vi "Configure Output.vi"(7 "Source Condition (2: Normal)":i32(ring)=2 items=["Zero", "HIZ", "Normal"], 8 "error in (no error)":errorcluster, 9 "Low Terminal State (1: Float)":i32(ring)=1 items=["Common", "Float"], 10 "Channel (1: Channel 1)":i32(ring)=1 items=["Channel 1"=1, "Channel 2"=2], 11 "VISA resource name":refnum<visa-resource-name>) -> (0 "error out":errorcluster, 3 "VISA resource name out":refnum<visa-resource-name>)   [LabVIEW 2017, in "Keysight B2980 Series.lvlib"]
doc: "Configures the low terminal and source condition for output.\n\n<b>Note(s):</b>\nThis VI is only applicable for model B2985A and B2987A."
uses:
  Keysight B2980 Series.lvlib
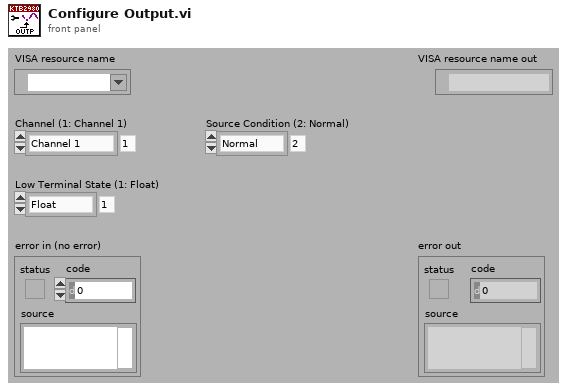
[diagram p1: front panel]
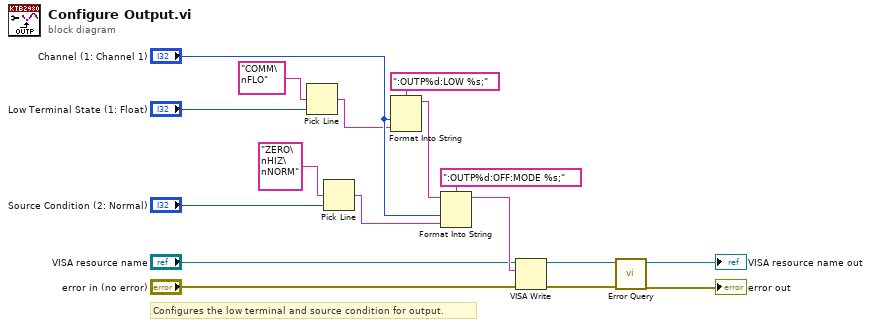
[diagram p0: block diagram]
diagram:
  # "Configures the low terminal and source condition for output."
  n1 = Pick Line(multi-line string="COMM\nFLO", line index="Low Terminal State (1: Float)") -> (output string=w13:string)  [unwired: 1 out]
  n2 = Pick Line(multi-line string="ZERO\nHIZ\nNORM", line index="Source Condition (2: Normal)") -> (output string=w8:string)  [unwired: 1 out]
  n3 = Format Into String(format string=":OUTP%d:LOW %s;", "Channel (1: Channel 1)", w13) -> (resulting string=w10:string)  [unwired: 2 in, 1 out]
  n4 = Format Into String(format string=":OUTP%d:OFF:MODE %s;", initial string=w10, "Channel (1: Channel 1)", w8) -> (resulting string=w7:string)  [unwired: 1 in, 1 out]
  n5 = VISA Write(VISA resource name="VISA resource name", write buffer=w7, error in (no error)="error in (no error)") -> (VISA resource name out=w4:refnum<visa-resource-name>, error out=w3:errorcluster)  [unwired: 1 out]
  n6 = call "Error Query.vi"("error in (no error)"=w3, "VISA resource name"=w4) -> ("error out"=→"error out":errorcluster, "VISA resource name out"=→"VISA resource name out":refnum<visa-resource-name>)  [unwired: 8 out]
